vi "or multiple inputs.vi"(2 "zero array in":dbl[](array[numeric]), 3 "input array in":bool[](array[boolean]), 4 "file data in":dbl[][](array[numeric])) -> (0 "array out":dbl[](array[numeric]), 1 "no input?":bool)   [LabVIEW 2014]
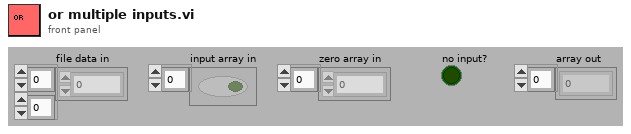
[diagram p1: front panel]
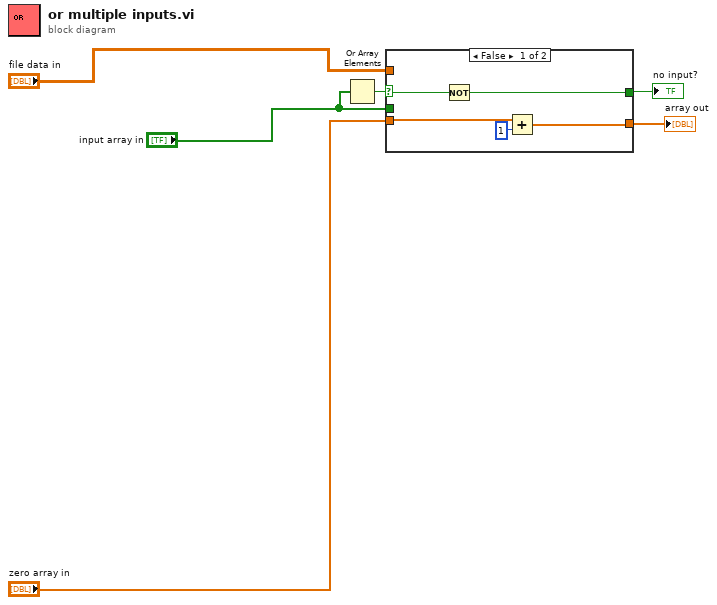
[diagram p0: block diagram]
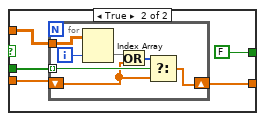
[diagram p2: hidden frame]
diagram:
  n1 = Or Array Elements(Boolean array="input array in") -> (logical OR=w4:bool)
  n2 = case shown="False" w4 {
    selector: w4 -> [w8 _]
    tunnel: "file data in" -> [_ w16]
    tunnel: "zero array in" -> [w11 w15]
    tunnel: "input array in" -> [_ w14]
    tunnel: [w9 w13] -> w3
    tunnel: [w7 FALSE] -> w6
    frame False {
      n3 = Not(x=w8) -> (.not. x?=w7:bool)
      n4 = Add(x=w11, y=1 ("element")) -> (x+y=w9:dbl[])
    }
    frame True {
      n5 = for {
        tunnel: w14 -> [w21] mode=indexing
        tunnel: w16 -> [w23]
        shift-right: [w17] -> w13
        shift-left: w15 -> [w18]
        i -> [w22]
        n6 = Index Array(array=w23, index (col)=w22) -> (element=w20:dbl[])  [unwired: 1 in]
        n7 = Or(x=w20, y=w18) -> (x .or. y?=w19:i32[])
        n8 = Select(t=w19, s=w21, f=w18) -> (s? t:f=w17:dbl[])
      }
    }
  }
  "no input?" <- w6
  "array out" <- w3
